vi "write_instr.vi"(4 "Range":T1(radio), 5 "Commands":string[](array[string]), 6 "Int. Bias (V)":dbl, 7 "Control Type":enum32{"User", "Photocap"}(tab), 8 "error in (no error)":errorcluster, 9 "Mode":enum32{"Cp", "Cs"}(radio), 10 "Zero Meter":bool, 11 "VISA In":refnum<visa-resource-name>) -> (0 "error out":errorcluster, 3 "VISA Out":refnum<visa-resource-name>)   [LabVIEW 2011]
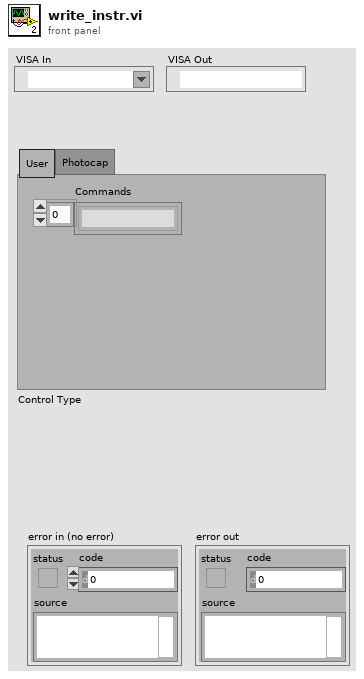
[diagram p1: front panel]
types:
  T1 = enum32{"2 pF/2 us", "20 pF/20 us", "200 pF/200 us", "2000 pF/2000 us", "Auto"}
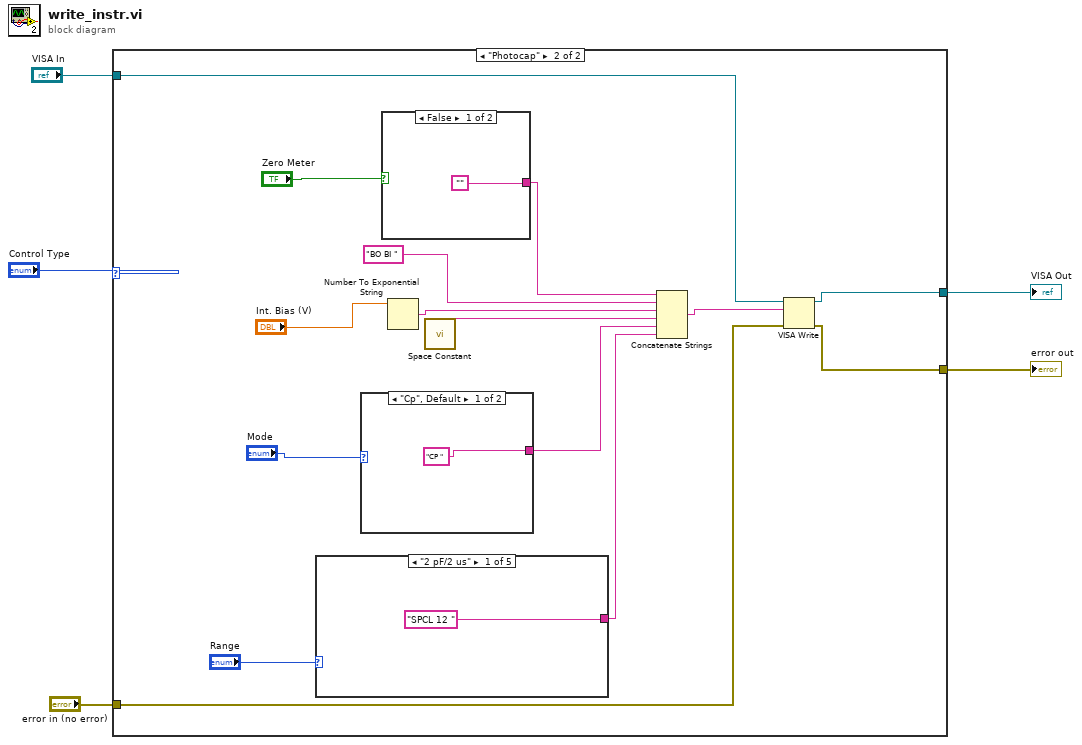
[diagram p0: block diagram]
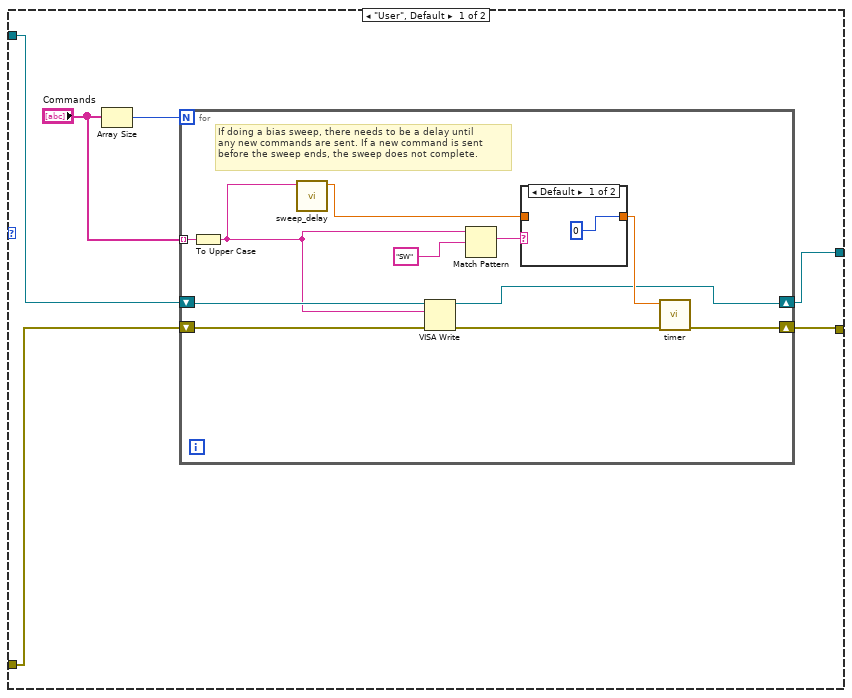
[diagram p2: hidden frame]
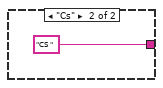
[diagram p4: hidden frame]
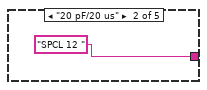
[diagram p5: hidden frame]
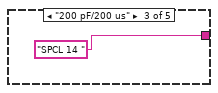
[diagram p6: hidden frame]
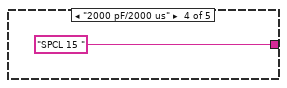
[diagram p7: hidden frame]
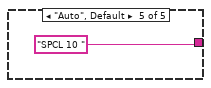
[diagram p8: hidden frame]
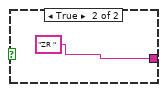
[diagram p9: hidden frame]
diagram:
  n1 = case shown="\"Photocap\"" "Control Type" {
    tunnel: "VISA In" -> [w7 w34]
    tunnel: "error in (no error)" -> [w6 w32]
    tunnel: [w9 w31] -> w2
    tunnel: [w8 w30] -> w1
    frame "User", Default {
      n2 = Array Size(array="Commands") -> (size(s)=w11:i32)
      n3 = for {
        N: w11 -> [_]
        shift-right: [w12] -> w9
        shift-left: w7 -> [w21]
        shift-right: [w13] -> w8
        shift-left: w6 -> [w22]
        tunnel: "Commands" -> [w14] mode=indexing
        # "If doing a bias sweep, there needs to be a delay until\nany new commands are sent. If a new command is sent\nbefore the sweep ends, the sweep does not complete."
        n4 = To Upper Case(1:w14) -> (0:w15:string)
        n5 = call "sweep_delay.vi"("Command"=w15) -> ("Delay Time"=w20:dbl)  [unwired: 10 in]
        n6 = VISA Write(VISA resource name=w21, write buffer=w15, error in (no error)=w22) -> (VISA resource name out=w12:refnum<visa-resource-name>, error out=w19:errorcluster)  [unwired: 1 out]
        n7 = Match Pattern(string=w15, regular expression="SW") -> (match substring=w17:string)  [unwired: 1 in, 3 out]
        n8 = case shown="Default" w17 {
          tunnel: w20 -> [_ w24]
          tunnel: [0 w24] -> w18
          frame Default {
          }
          frame "SW" {
          }
        }
        n9 = call "timer.vi"("error in (no error)"=w19, "Delay Time"=w18) -> ("error out"=w13:errorcluster)  [unwired: 9 in]
      }
    }
    frame "Photocap" {
      n10 = case shown="\"2 pF/2 us\"" "Range" {
        tunnel: ["SPCL 12 " "SPCL 12 " "SPCL 14 " "SPCL 15 " "SPCL 10 "] -> w35
        frame "2 pF/2 us" {
        }
        frame "20 pF/20 us" {
        }
        frame "200 pF/200 us" {
        }
        frame "2000 pF/2000 us" {
        }
        frame "Auto", Default {
        }
      }
      n11 = case shown="\"Cp\", Default" "Mode" {
        tunnel: ["CP " "CS "] -> w29
        frame "Cp", Default {
        }
        frame "Cs" {
        }
      }
      n12 = case shown="False" "Zero Meter" {
        tunnel: ["" "ZR "] -> w25
        frame False {
        }
        frame True {
        }
      }
      n13 = Number To Exponential String(number="Int. Bias (V)") -> (E-format string=w27:string)  [unwired: 3 in]
      n14 = call <vilib>:"Space Constant.vi"() -> ("String"=w28:string)
      n15 = Concatenate Strings(w25, "BO BI ", w27, w28, w29, w35) -> (w33:string)
      n16 = VISA Write(VISA resource name=w34, write buffer=w33, error in (no error)=w32) -> (VISA resource name out=w31:refnum<visa-resource-name>, error out=w30:errorcluster)  [unwired: 1 out]
    }
  }
  "error out" <- w1
  "VISA Out" <- w2
